vi "GetMatlabCOM_FingerPressRT.vi"(1 "MatlabCOM":string, 2 "Mode":enum16{"Initialize", "Run"}(ring)) -> (0 "ParsedCOM":T1)   [LabVIEW 2011]
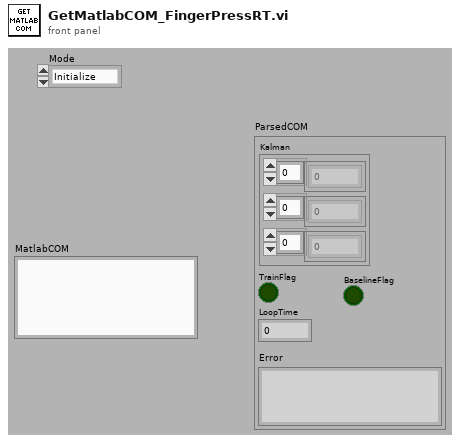
[diagram p1: front panel]
types:
  T1 = cluster{"Kalman":cluster{dbl[], dbl[], dbl[]}, "TrainFlag":bool, "LoopTime":dbl, "Error":string, "BaselineFlag":bool}
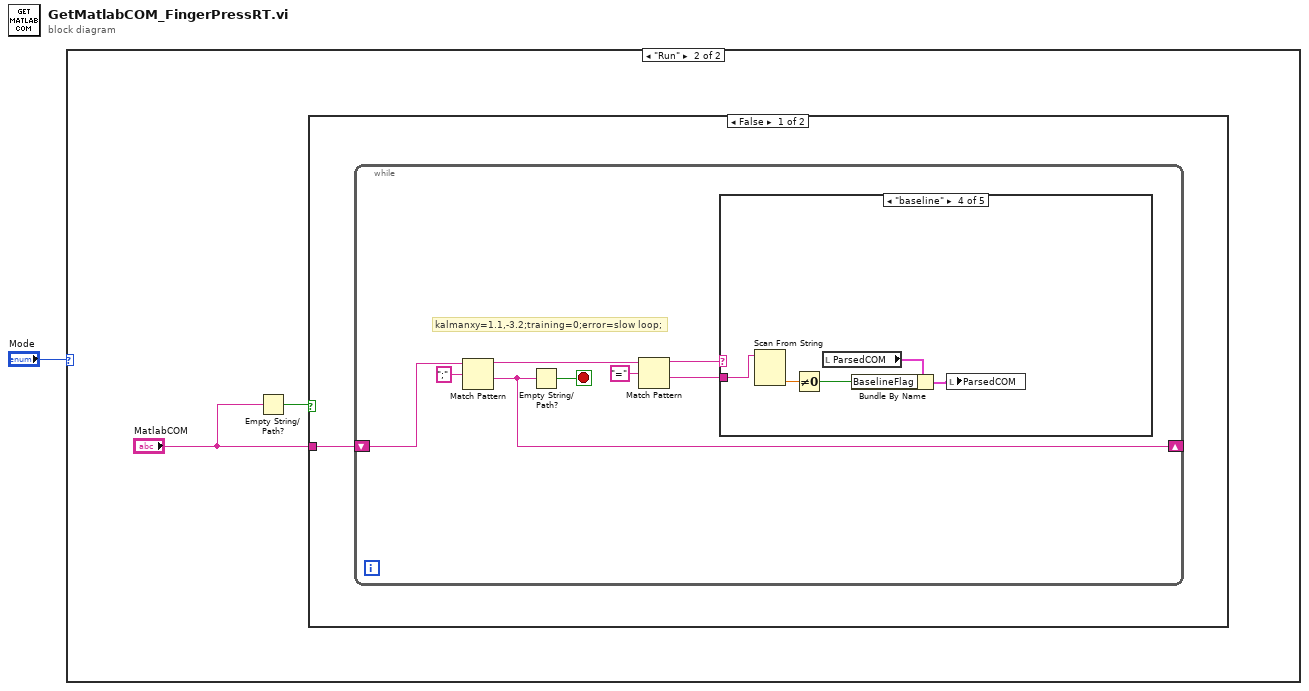
[diagram p0: block diagram]
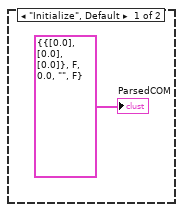
[diagram p2: hidden frame]
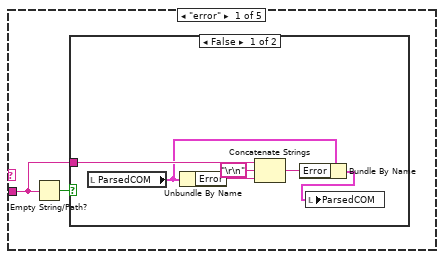
[diagram p3: hidden frame]
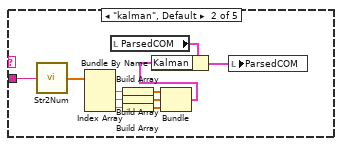
[diagram p5: hidden frame]
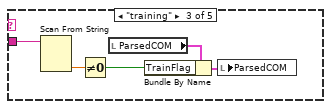
[diagram p6: hidden frame]
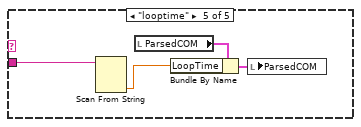
[diagram p7: hidden frame]
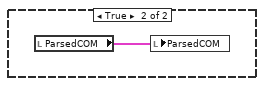
[diagram p8: hidden frame]
diagram:
  n1 = case shown="\"Run\"" "Mode" {
    frame "Initialize", Default {
      "ParsedCOM" <- T1 {"Kalman"={[0.0], [0.0], [0.0]}, "TrainFlag"=FALSE, "LoopTime"=0.0, "Error"="", "BaselineFlag"=FALSE} ("ParsedCOM")
    }
    frame "Run" {
      n2 = Empty String/Path?(string/path="MatlabCOM") -> (empty?=w3:bool)
      n3 = case shown="False" w3 {
        tunnel: "MatlabCOM" -> [w5 _]
        frame False {
          n4 = while {
            shift-right: [w10] -> _
            shift-left: w5 -> [w11]
            stop <- w12 stop-if-true
            # "kalmanxy=1.1,-3.2;training=0;error=slow loop;"
            n5 = Match Pattern(string=w11, regular expression=";") -> (before substring=w9:string, after substring=w10:string)  [unwired: 1 in, 2 out]
            n6 = Empty String/Path?(string/path=w10) -> (empty?=w12:bool)
            n7 = Match Pattern(string=w9, regular expression="=") -> (before substring=w7:string, after substring=w6:string)  [unwired: 1 in, 2 out]
            n8 = case shown="\"baseline\"" w7 {
              tunnel: w6 -> [w14 w32 w36 w38 w46]
              frame "error" {
                n9 = Empty String/Path?(string/path=w14) -> (empty?=w15:bool)
                n10 = case shown="False" w15 {
                  tunnel: w14 -> [w20 _]
                  frame False {
                    n11 = local read "ParsedCOM"() -> (w19:T1)
                    n12 = Unbundle By Name(w19) -> ("Error"=w17:string)
                    n13 = Concatenate Strings(w20, "\r\n", w17) -> (w16:string)
                    n14 = Bundle By Name(cluster=w19, "Error"=w16) -> (w21:T1)
                    n15 = local write "ParsedCOM"(w21) -> ()
                  }
                  frame True {
                  }
                }
              }
              frame "kalman", Default {
                n16 = call "Str2Num.vi"("InputString"=w32) -> ("Array"=w25:dbl[])
                n17 = Index Array(array=w25) -> (element #1=w29:dbl, element #2=w28:dbl, element #3=w24:dbl)  [unwired: 3 in]
                n18 = local read "ParsedCOM"() -> (w31:T1)
                n19 = Build Array(w29) -> (w27:dbl[])
                n20 = Build Array(w28) -> (w26:dbl[])
                n21 = Build Array(w24) -> (w23:dbl[])
                n22 = Bundle(w27, w26, w23) -> (w22:cluster{dbl[], dbl[], dbl[]})  [unwired: 1 in]
                n23 = Bundle By Name(cluster=w31, "Kalman"=w22) -> (w30:T1)
                n24 = local write "ParsedCOM"(w30) -> ()
              }
              frame "training" {
                n25 = Scan From String(input string=w36) -> (output 1=w34:dbl)  [unwired: 4 in, 3 out]
                n26 = Not Equal To 0?(x=w34) -> (x != 0?=w33:bool)
                n27 = local read "ParsedCOM"() -> (w37:T1)
                n28 = Bundle By Name(cluster=w37, "TrainFlag"=w33) -> (w35:T1)
                n29 = local write "ParsedCOM"(w35) -> ()
              }
              frame "baseline" {
                n30 = Scan From String(input string=w38) -> (output 1=w40:dbl)  [unwired: 4 in, 3 out]
                n31 = Not Equal To 0?(x=w40) -> (x != 0?=w39:bool)
                n32 = local read "ParsedCOM"() -> (w42:T1)
                n33 = Bundle By Name(cluster=w42, "BaselineFlag"=w39) -> (w41:T1)
                n34 = local write "ParsedCOM"(w41) -> ()
              }
              frame "looptime" {
                n35 = Scan From String(input string=w46) -> (output 1=w43:dbl)  [unwired: 4 in, 3 out]
                n36 = local read "ParsedCOM"() -> (w45:T1)
                n37 = Bundle By Name(cluster=w45, "LoopTime"=w43) -> (w44:T1)
                n38 = local write "ParsedCOM"(w44) -> ()
              }
            }
          }
        }
        frame True {
          n39 = local read "ParsedCOM"() -> (w47:T1)
          n40 = local write "ParsedCOM"(w47) -> ()
        }
      }
    }
  }
